vi "Out_S9F5.vi"(8 "error in (no error)":errorcluster, 10 "Message Header":u8[](array[numeric]), 11 "S9 Message Class in":refnum<class "S9 Message Class.lvclass">) -> (0 "error out":errorcluster, 3 "S9 Message Class out":refnum<class "S9 Message Class.lvclass">)   [LabVIEW 2020, in "SECS Communication.lvlib" / "S9 Message Class.lvclass"]
uses:
  S9 Message Class.lvclass
  D:/Dropbox/SECS/LabVIEW Code/Com/SECS Communication/SECS-II Class/SECS-II Class.lvclass
  SECS-II Class/Data Message_Binary.vi
  S9 Message Class.lvclass/S9 Message Class.ctl
  SECS-II Class/SECS-II Class.lvclass
  D:/Dropbox/SECS/LabVIEW Code/Com/SECS Communication/S9 Message Class/S9 Message Class.lvclass
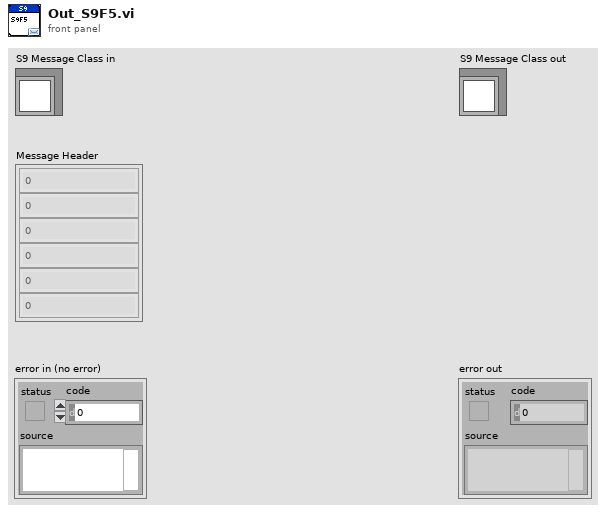
[diagram p1: front panel]
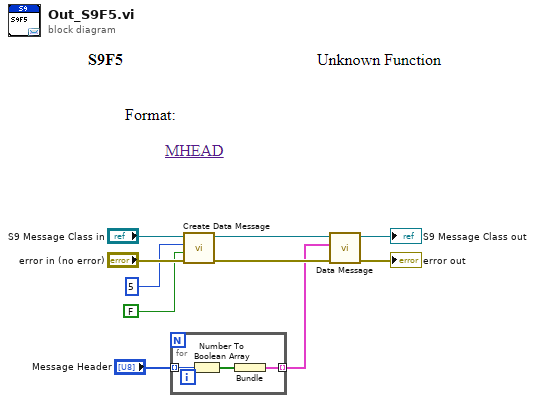
[diagram p0: block diagram]
diagram:
  n1 = for {
    tunnel: "Message Header" -> [w13] mode=indexing
    tunnel: [w11] -> w3 mode=indexing
    n2 = Number To Boolean Array(number=w13) -> (Boolean array=w12:bool[])
    n3 = Bundle("Boolean array"=w12) -> (w11:cluster{"Boolean array":bool[]})  [unwired: 1 in]
  }
  n4 = call "Create Data Message.vi"("error in (no error)"="error in (no error)", "W-Bit"=FALSE, "Function"=u8 5, "SECS-II Class in"="S9 Message Class in") -> ("error out"=w6:errorcluster, "SECS-II Class out"=w5:refnum<class "S9 Message Class.lvclass">)  [unwired: 6 in]
  n5 = call-poly "Data Message.vi"("error in"=w6, "Data Cluster"=w3, "SECS-II Class in"=w5) -> ("error out"=→"error out":errorcluster, "SECS-II Class out"=→"S9 Message Class out":refnum<class "S9 Message Class.lvclass">)  [unwired: 7 in]
